vi "Do.vi"(8 "error in":errorcluster, 10 "Actor in":refnum<class "Actor.lvclass">, 11 "DS Reply Msg in":refnum<class "DS Reply Msg.lvclass">) -> (0 "error out":errorcluster, 2 "Actor out":refnum<class "Actor.lvclass">)   [LabVIEW 2023, in "DS Reply Msg.lvclass"]
uses:
  DS Reply Msg.lvclass
  <vilib>/ActorFramework/Actor/Actor.lvclass
  DS Reply Msg.lvclass/DS Reply Msg.ctl
panel:
  in  "1122 error message":string="This actor was sent a Reply Msg. The sender set a time out duration. While this actor worked on the message, the sender timed out, resulting in this error. The Actor Framework cannot specify further what should happen; that is a policy decision that must be made by this actor. In most cases, programmers will override either this message's Do.vi or this actor's Handle Error.vi to throw away the computed result and clear this error, but some actors may do more sophisticated work (such as going ahead and sending the result to the sender in a separate asynchronous message)."
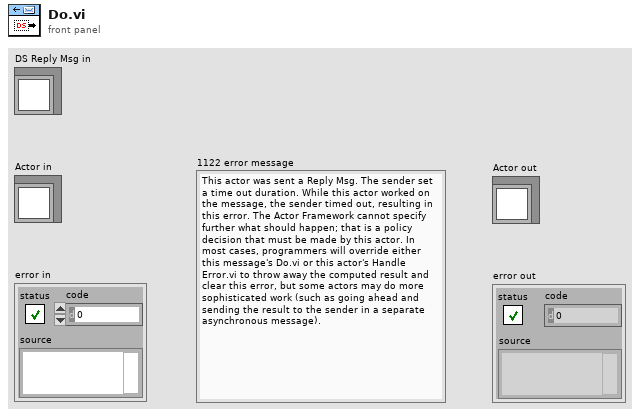
[diagram p1: front panel]
types:
  T1 = enum16{"Read", "Write", "ReadWrite", "BufferedRead", "BufferedReadWrite"}
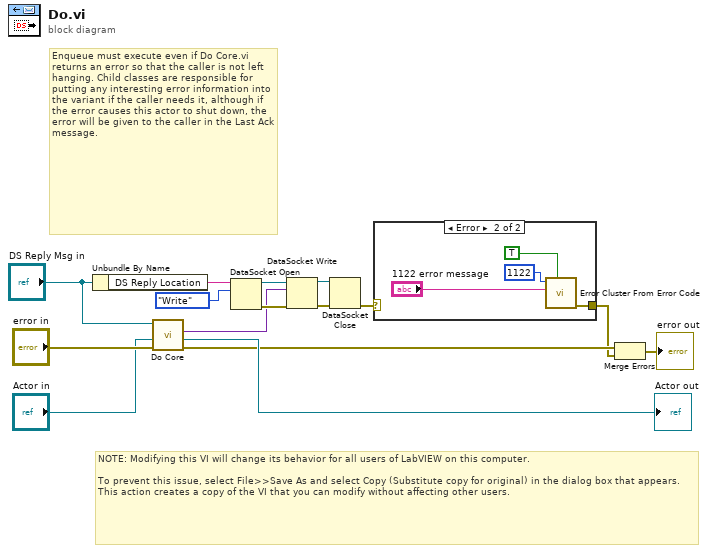
[diagram p0: block diagram]
diagram:
  # "Enqueue must execute even if Do Core.vi returns an error so that the caller is not left hanging. Child classes are responsible for putting any interesting error information into the variant if the caller needs it, although if the error causes this actor to shut down, the error will be given to the caller in the Last Ack message."
  # "NOTE: Modifying this VI will change its behavior for all users of LabVIEW on this computer.\n\nTo prevent this issue, select File>>Save As and select Copy (Substitute copy for original) in the dialog box that appears. This action creates a copy of the VI that you can modify without affecting other users."
  n1 = Unbundle By Name("DS Reply Msg in") -> ("DS Reply Location"=w4:string)
  n2 = call-dynamic "Do Core.vi"("error in"="error in", "Actor in"="Actor in", "DS Reply Msg in"="DS Reply Msg in") -> ("error out"=w11:errorcluster, "Actor out"=→"Actor out":refnum<class "Actor.lvclass">, "Reply"=w1:variant)  [unwired: 6 in]
  n3 = DataSocket Open(10:T1."Write" ("mode"), 11:w4) -> (0:w7:errorcluster, 3:w8:refnum<k13>)  [unwired: 2 in]
  n4 = DataSocket Write(8:w7, 10:w1, 11:w8) -> (0:w9:errorcluster, 3:w2:refnum<k13>)  [unwired: 2 out]
  n5 = DataSocket Close(8:w9, 11:w2) -> (0:w3:errorcluster)  [unwired: 1 in, 1 out]
  n6 = case shown="Error" w3 {
    selector: w3 -> [w16 _]
    tunnel: [w16 w17] -> w10
    frame No Error {
    }
    frame Error {
      n7 = call <vilib>:"Error Cluster From Error Code.vi"("show call chain? (False)"=TRUE, "error message (\"\")"="1122 error message", "error code (0)"=1122) -> ("error out"=w17:errorcluster)  [unwired: 6 in]
    }
  }
  n8 = Merge Errors(w11, w10) -> (→"error out":errorcluster)
